vi "FTW-Actor.vi"(0 "FTW Actor Instance":refnum<class "FTW-ActorInstance.lvclass">, 5 "FTW Actor Instance Configuration":string="{\n  \"Identity\": \"ActorName\",\n  \"InboxAddress\": \"inproc://*\",\n  \"LoggerAddress\": \"\",\n  \"DebugEnableInboxLogging\": false,\n  \"DebugEnableJobLogging\": false,\n  \"LauncherAddress\": \"\"\n}", 11 "ErrorIn":errorcluster) -> (15 "Error":errorcluster)   [LabVIEW 2015, in "FTW-ActorInstance.lvclass"]
uses:
  FTW-ActorInstance.lvclass
  Message/Base/FTW-Message.lvclass
  FTW-ActorInstance.lvclass/FTW-ActorInstance.ctl
  JobSequencer/FTW-SEQ-Current.vi
  Message/Request/FTW-Message-IncomingRequest.lvclass
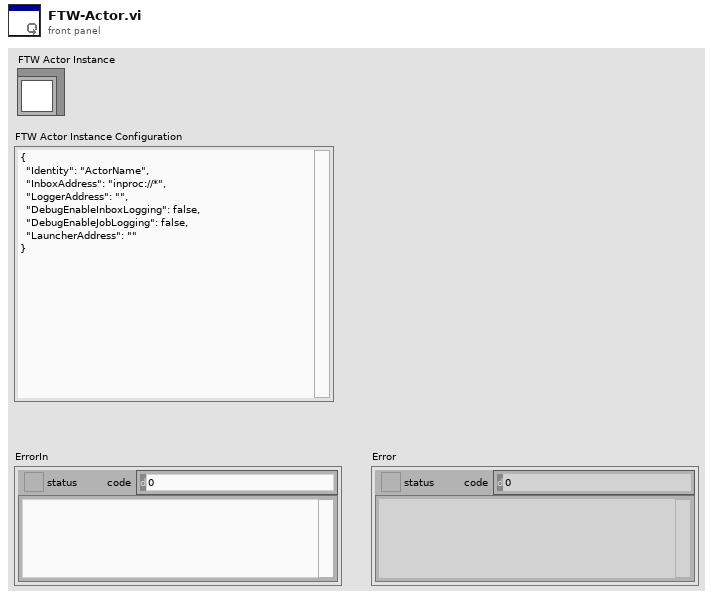
[diagram p1: front panel]
types:
  T1 = cluster{"Incoming Requests":refnum<event-registration>, "Local Messages":refnum<event-registration>, "Additional Registration Types":refnum<event-registration>}
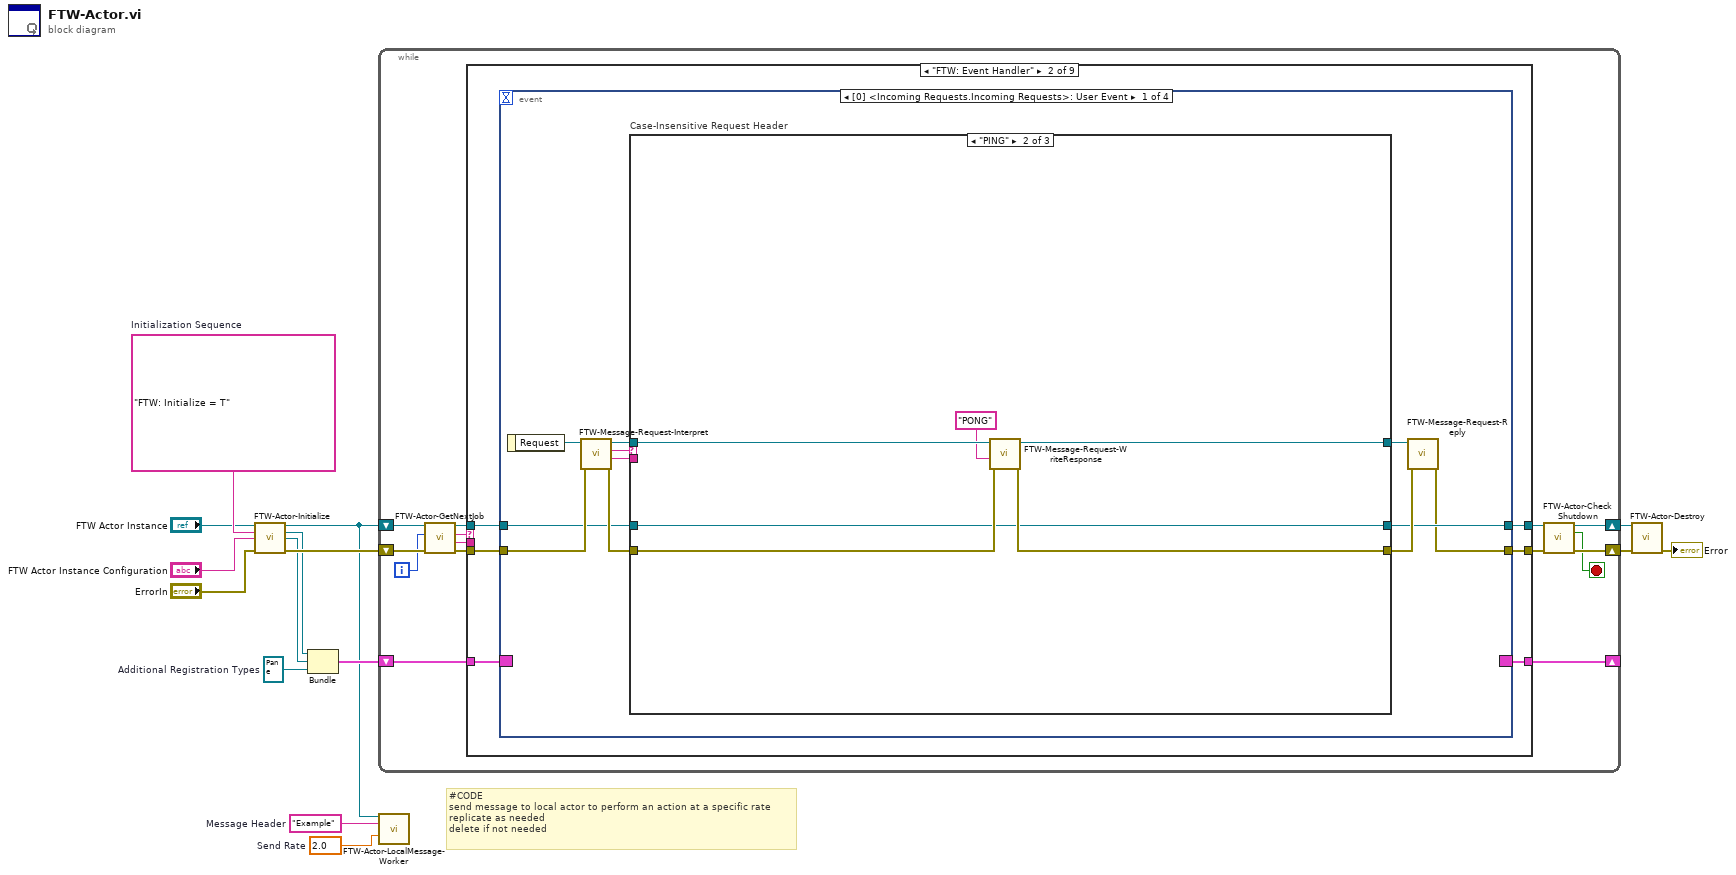
[diagram p0: block diagram]
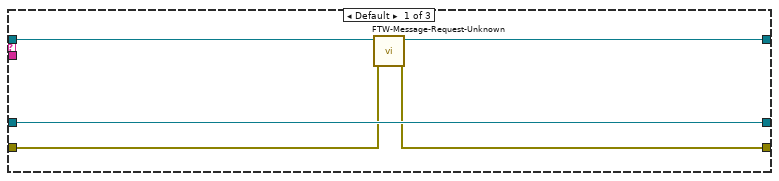
[diagram p3: hidden frame]
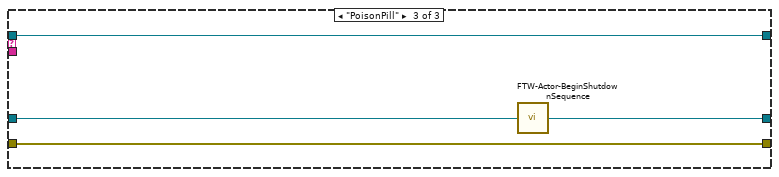
[diagram p4: hidden frame]
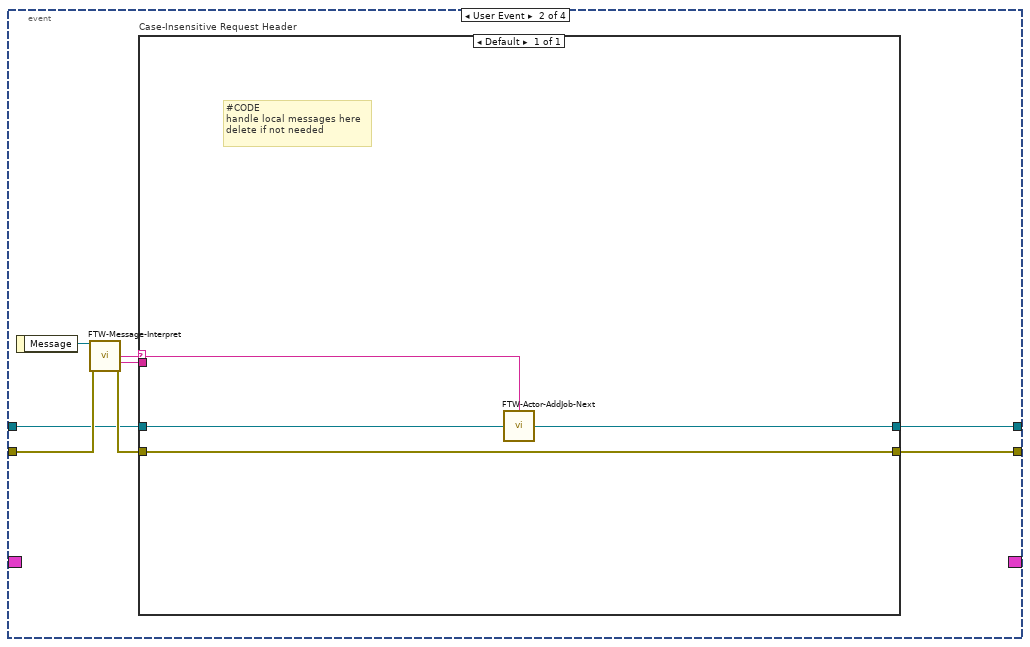
[diagram p5: hidden frame]
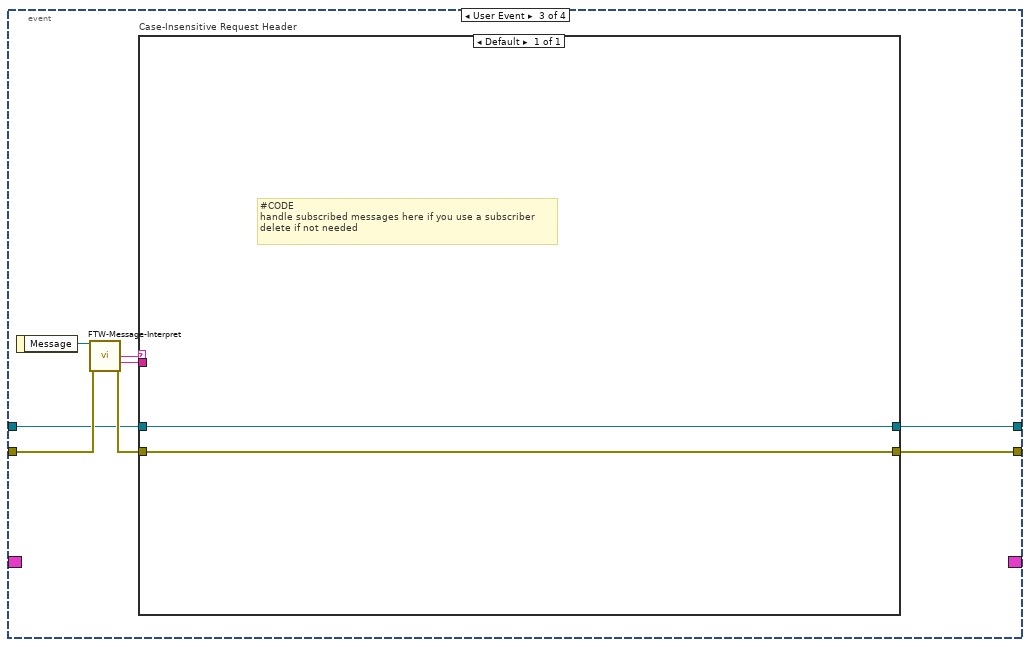
[diagram p6: hidden frame]
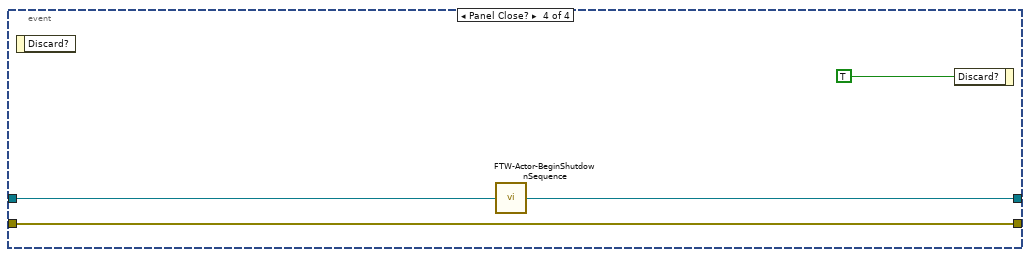
[diagram p7: hidden frame]
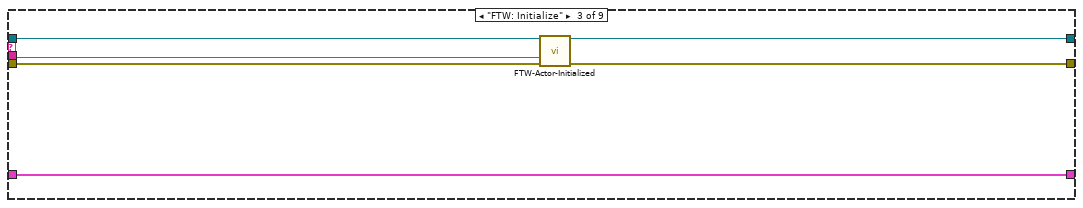
[diagram p8: hidden frame]
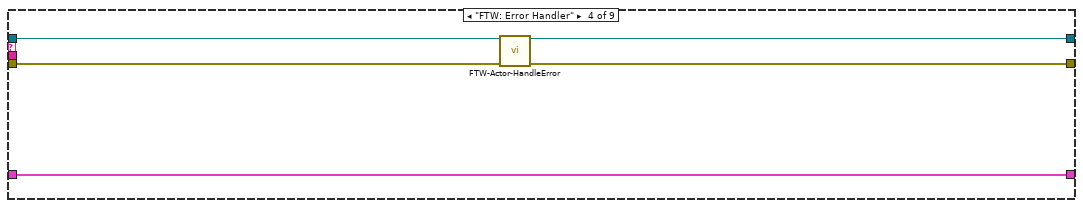
[diagram p9: hidden frame]
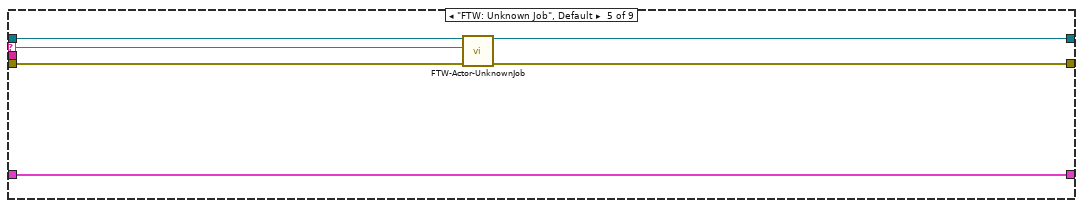
[diagram p10: hidden frame]
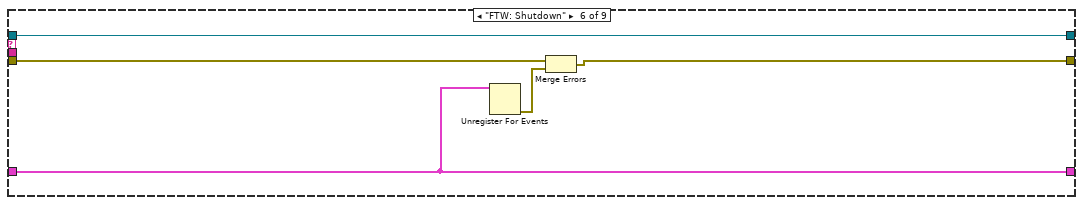
[diagram p11: hidden frame]
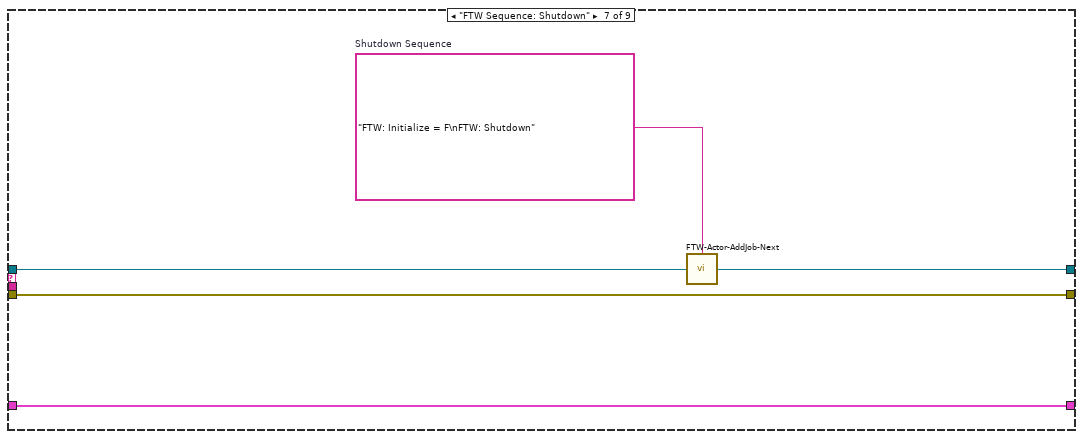
[diagram p12: hidden frame]
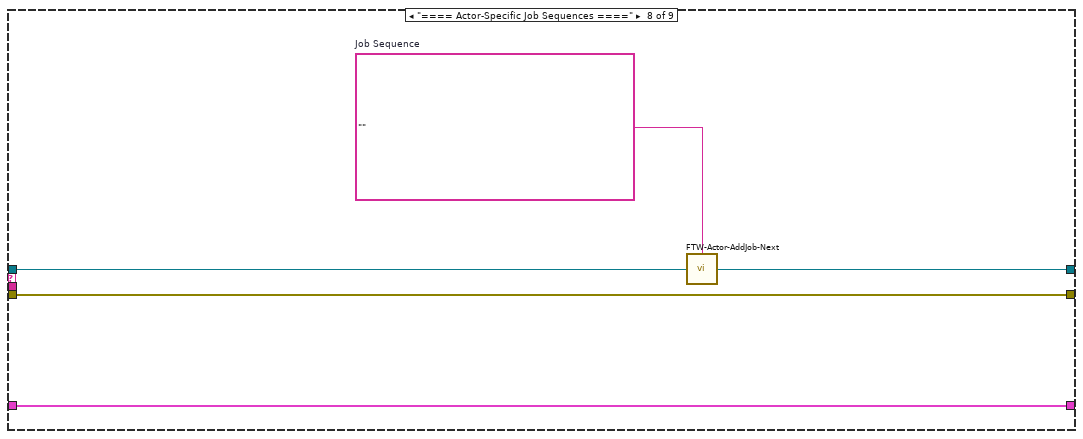
[diagram p13: hidden frame]
diagram:
  w2 = 2.0  # Send Rate
  w3 = "Example"  # Message Header
  w5 = refnum<event-registration> refnum  # Additional Registration Types
  w11 = "FTW: Initialize = T"  # Initialization Sequence
  # "#CODE\nsend message to local actor to perform an action at a specific rate\nreplicate as needed\ndelete if not needed"
  n1 = call-dynamic "FTW-Actor-Initialize.vi"("FTW Actor Instance Type"="FTW Actor Instance", "Initialization Job Sequence"=w11, "Actor Instance Configuration"="FTW Actor Instance Configuration", "error in"="ErrorIn") -> ("FTW Actor Instance"=w4:refnum<class "FTW-ActorInstance.lvclass">, "Incoming Requests"=w7:refnum<event-registration>, "Local Messages"=w6:refnum<event-registration>, "error out"=w12:errorcluster)  [unwired: 8 in]
  n2 = Bundle("Incoming Requests"=w7, "Local Messages"=w6, "Additional Registration Types"=w5) -> (w9:T1)  [unwired: 1 in]
  n3 = while {
    shift-right: [w19] -> w14
    shift-left: w12 -> [w26]
    shift-right: [w16] -> _
    shift-left: w9 -> [w29]
    shift-right: [w21] -> w15
    shift-left: w4 -> [w28]
    i -> [w17]
    stop <- w18 stop-if-true
    n4 = call "FTW-Actor-GetNextJob.vi"("error in"=w26, "Jobs Performed"=w17, "FTW Actor Instance"=w28) -> ("error out"=w25:errorcluster, "Job Data"=w23:string, "Job Name"=w24:string, "FTW Actor Instance out"=w27:refnum<class "FTW-ActorInstance.lvclass">)  [unwired: 5 in]
    n5 = case shown="\"FTW: Event Handler\"" w24 {
      selector: w24 -> [_ _ _ _ w102 _ _ _ _]
      tunnel: [w31 w38 w92 w97 w105 w111 w116 w121 w125] -> w20
      tunnel: w25 -> [w31 w37 w95 w99 w106 w112 w116 w121 w125]
      tunnel: w29 -> [w32 w33 w96 w101 w107 w108 w117 w122 w124]
      tunnel: [w32 w36 w96 w101 w107 w108 w117 w122 w124] -> w16
      tunnel: w23 -> [_ _ w91 _ _ _ _ _ _]
      tunnel: [w30 w35 w93 w98 w103 w109 w114 w119 w123] -> w22
      tunnel: w27 -> [w30 w34 w94 w100 w104 w109 w115 w120 w123]
      frame "==== Featherweight Framework Jobs ====" {
      }
      frame "FTW: Event Handler" {
        n6 = event shown="[0] <Incoming Requests.Incoming Requests>: User Event" {
          selector: w33 -> [_ _ _ _]
          dyn-events: [_ _ _ _] -> w36
          timeout: _ -> [_ _ _ _]
          tunnel: [w41 w69 w81 w89] -> w38
          tunnel: w37 -> [w47 w70 w82 w89]
          tunnel: [w45 w68 w80 w87] -> w35
          tunnel: w34 -> [w44 w67 w79 w88]
          event User Event {
            n7 = event-data() -> ("Request"=w48:refnum<class "FTW-Message-IncomingRequest.lvclass">)  [unwired: 1 in]
            n8 = call "FTW-Message-Request-Interpret.vi"("error in"=w47, "FTW Incoming Request"=w48) -> ("error out"=w49:errorcluster, "Request Body"=w39:string, "Request Header"=w43:string, "FTW Incoming Request out"=w42:refnum<class "FTW-Message-IncomingRequest.lvclass">)  [unwired: 6 in]
            n9 = case "Case-Insensitive Request Header" shown="\"PING\"" w43 {
              tunnel: [w52 w58 w63] -> w46
              tunnel: w49 -> [w53 w59 w63]
              tunnel: [w54 w57 w64] -> w45
              tunnel: w44 -> [w54 w57 w62]
              tunnel: w42 -> [w51 w60 w61]
              tunnel: [w50 w56 w61] -> w40
              tunnel: w39 -> [_ _ _]
              frame Default {
                n10 = call "FTW-Message-Request-Unknown.vi"("error in"=w53, "FTW Incoming Request"=w51) -> ("error out"=w52:errorcluster, "FTW Incoming Request Out"=w50:refnum<class "FTW-Message-IncomingRequest.lvclass">)  [unwired: 8 in]
              }
              frame "PING" {
                n11 = call "FTW-Message-Request-WriteResponse.vi"("error in"=w59, "Response Body"="PONG" ("Response Header"), "FTW Incoming Request"=w60) -> ("error out"=w58:errorcluster, "FTW Incoming Request out"=w56:refnum<class "FTW-Message-IncomingRequest.lvclass">)  [unwired: 7 in]
              }
              frame "PoisonPill" {
                n12 = call "FTW-Actor-BeginShutdownSequence.vi"("FTW Actor Instance"=w62) -> ("FTW Actor Instance out"=w64:refnum<class "FTW-ActorInstance.lvclass">)  [unwired: 3 in]
              }
            }
            n13 = call "FTW-Message-Request-Reply.vi"("FTW: Reply Error"=w46, "FTW Incoming Request"=w40) -> ("error out"=w41:errorcluster)  [unwired: 8 in, 1 out]
          }
          event User Event {
            n14 = event-data() -> ("Message"=w71:refnum<class "FTW-Message.lvclass">)  [unwired: 1 in]
            n15 = call-dynamic "FTW-Message-Interpret.vi"("FTW Message"=w71, "error in"=w70) -> ("Message Header"=w65:string, "Message Body"=w66:string, "error out"=w72:errorcluster)  [unwired: 9 in, 2 out]
            n16 = case "Case-Insensitive Request Header" shown="Default" w65 {
              selector: w65 -> [w73]
              tunnel: [w75] -> w69
              tunnel: w72 -> [w75]
              tunnel: [w74] -> w68
              tunnel: w67 -> [w76]
              tunnel: w66 -> [_]
              frame Default {
                # "#CODE\nhandle local messages here\ndelete if not needed"
                n17 = call "FTW-Actor-AddJob-Next.vi"("Add Next in Job Queue"=w73, "FTW Actor Instance"=w76) -> ("FTW Actor Instance out"=w74:refnum<class "FTW-ActorInstance.lvclass">)  [unwired: 2 in]
              }
            }
          }
          event User Event {
            n18 = event-data() -> ("Message"=w83:refnum<class "FTW-Message.lvclass">)  [unwired: 1 in]
            n19 = call-dynamic "FTW-Message-Interpret.vi"("FTW Message"=w83, "error in"=w82) -> ("Message Header"=w77:string, "Message Body"=w78:string, "error out"=w84:errorcluster)  [unwired: 9 in, 2 out]
            n20 = case "Case-Insensitive Request Header" shown="Default" w77 {
              tunnel: [w85] -> w81
              tunnel: w84 -> [w85]
              tunnel: [w86] -> w80
              tunnel: w79 -> [w86]
              tunnel: w78 -> [_]
              frame Default {
                # "#CODE\nhandle subscribed messages here if you use a subscriber\ndelete if not needed"
              }
            }
          }
          event Panel Close? {
            n21 = event-data() -> ()  [unwired: 1 in, 1 out]
            n22 = call "FTW-Actor-BeginShutdownSequence.vi"("FTW Actor Instance"=w88) -> ("FTW Actor Instance out"=w87:refnum<class "FTW-ActorInstance.lvclass">)  [unwired: 3 in]
            n23 = event-data("Discard?"=TRUE) -> ()  [unwired: 1 in, 1 out]
          }
        }
      }
      frame "FTW: Initialize" {
        n24 = call-dynamic "FTW-Actor-Initialized.vi"("FTW Actor Instance"=w94, "Positive Init?"=w91, "error in"=w95) -> ("FTW Actor Instance out"=w93:refnum<class "FTW-ActorInstance.lvclass">, "error out"=w92:errorcluster)  [unwired: 11 in]
      }
      frame "FTW: Error Handler" {
        n25 = call-dynamic "FTW-Actor-HandleError.vi"("FTW Actor Instance"=w100, "error in"=w99) -> ("FTW Actor Instance out"=w98:refnum<class "FTW-ActorInstance.lvclass">, "error out"=w97:errorcluster)  [unwired: 10 in, 2 out]
      }
      frame "FTW: Unknown Job", Default {
        n26 = call-dynamic "FTW-Actor-UnknownJob.vi"("FTW Actor Instance"=w104, "Unknown Job"=w102, "error in"=w106) -> ("FTW Actor Instance out"=w103:refnum<class "FTW-ActorInstance.lvclass">, "error out"=w105:errorcluster)  [unwired: 11 in]
      }
      frame "FTW: Shutdown" {
        n27 = Unregister For Events(event registration refnum=w108) -> (error out=w110:errorcluster)  [unwired: 1 in]
        n28 = Merge Errors(w112, w110) -> (w111:errorcluster)
      }
      frame "FTW Sequence: Shutdown" {
        w113 = "FTW: Initialize = F\nFTW: Shutdown"  # Shutdown Sequence
        n29 = call "FTW-Actor-AddJob-Next.vi"("Add Next in Job Queue"=w113, "FTW Actor Instance"=w115) -> ("FTW Actor Instance out"=w114:refnum<class "FTW-ActorInstance.lvclass">)  [unwired: 2 in]
      }
      frame "==== Actor-Specific Job Sequences ====" {
        w118 = ""  # Job Sequence
        n30 = call "FTW-Actor-AddJob-Next.vi"("Add Next in Job Queue"=w118, "FTW Actor Instance"=w120) -> ("FTW Actor Instance out"=w119:refnum<class "FTW-ActorInstance.lvclass">)  [unwired: 2 in]
      }
      frame "==== Actor-Specific Jobs ====" {
      }
    }
    n31 = call "FTW-Actor-CheckShutdown.vi"("FTW Actor Instance"=w22, "error in"=w20) -> ("FTW Actor Instance out"=w21:refnum<class "FTW-ActorInstance.lvclass">, "Shutdown?"=w18:bool, "error out"=w19:errorcluster)  [unwired: 11 in]
  }
  n32 = call-dynamic "FTW-Actor-LocalMessage-Worker.vi"("FTW-ActorInstance In"=w4, "Message Header"=w3, "Send Rate"=w2) -> ()  [unwired: 13 in]
  n33 = call-dynamic "FTW-Actor-Destroy.vi"("FTW Actor Instance"=w15, "error in"=w14) -> ("error out"=→"Error":errorcluster)  [unwired: 13 in]
